vi "GDFeventTypeHandler.vi"(1 "EventTypeCode":u16) -> (0 "EventTypeString":string)   [LabVIEW 2016, in "GDF File Reader.lvlib"]
uses:
  GDF File Reader.lvlib
panel:
  # "This VI is a part of BCI Design library, http://www.ru-bci.org \nCopyright © 2020, Sotnikov Peter, All rights reserved. License: CC BY-NC 4.0"
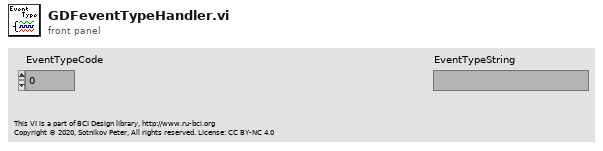
[diagram p1: front panel]
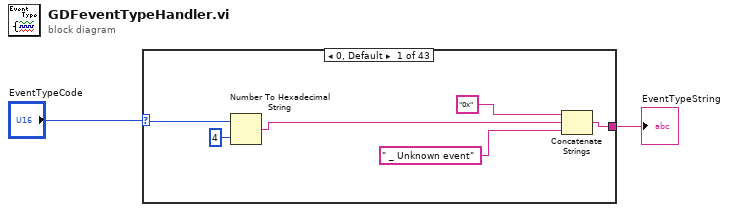
[diagram p0: block diagram]
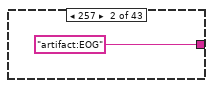
[diagram p2: hidden frame]
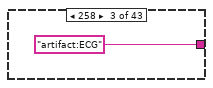
[diagram p3: hidden frame]
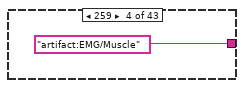
[diagram p4: hidden frame]
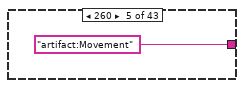
[diagram p5: hidden frame]
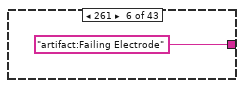
[diagram p6: hidden frame]
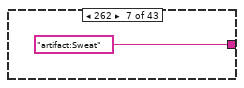
[diagram p7: hidden frame]
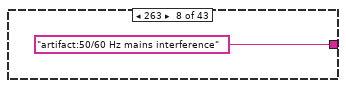
[diagram p8: hidden frame]
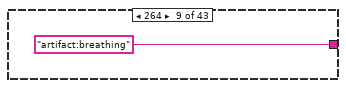
[diagram p9: hidden frame]
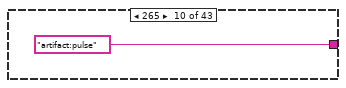
[diagram p10: hidden frame]
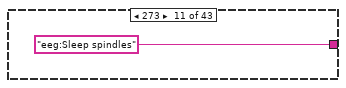
[diagram p11: hidden frame]
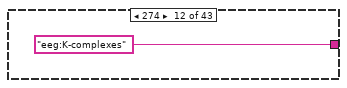
[diagram p12: hidden frame]
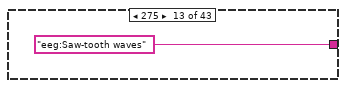
[diagram p13: hidden frame]
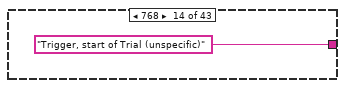
[diagram p14: hidden frame]
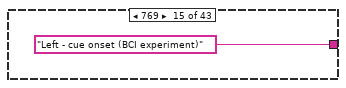
[diagram p15: hidden frame]
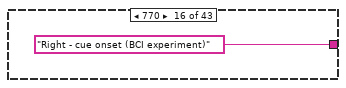
[diagram p16: hidden frame]
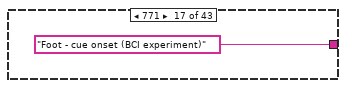
[diagram p17: hidden frame]
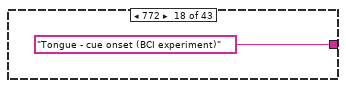
[diagram p18: hidden frame]
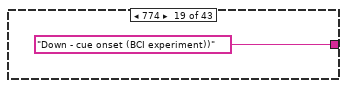
[diagram p19: hidden frame]
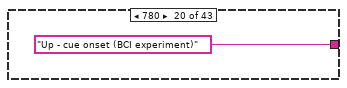
[diagram p20: hidden frame]
diagram:
  n1 = case shown="0, Default" "EventTypeCode" {
    selector: "EventTypeCode" -> [w7 _ _ _ _ _ _ _ _ _ _ _ _ _ _ _ _ _ _ _ _ _ _ _ _ _ _ _ _ _ _ _ _ _ _ _ _ _ _ _ _ _ _]
    tunnel: [w6 "artifact:EOG" "artifact:ECG" "artifact:EMG/Muscle" "artifact:Movement" "artifact:Failing Electrode" "artifact:Sweat" "artifact:50/60 Hz mains interference" "artifact:breathing" "artifact:pulse" "eeg:Sleep spindles" "eeg:K-complexes" "eeg:Saw-tooth waves" "Trigger, start of Trial (unspecific)" "Left - cue onset (BCI experiment)" "Right - cue onset (BCI experiment)" "Foot - cue onset (BCI experiment)" "Tongue - cue onset (BCI experiment)" "Down - cue onset (BCI experiment))" "Up - cue onset (BCI experiment)" "Feedback (continuous) - onset (BCI experiment)" "Feedback (discrete) - onset (BCI experiment)" "Beep (accustic stimulus, BCI experiment)" "Cross on screen (BCI experiment)" "Rejection of whole trial" "Obstructive Apnea/Hypopnea Event (OAHE)" "Respiratory Effort Related Arousal (RERA)" "Central Apnea/Hypopnea Event (CAHE)" "Cheyne-Stokes Breathing (CSB)" "Sleep Hypoventilation" "Wake" "Stage 1" "Stage 2" "Stage 3" "Stage 4" "REM" "ecg:Fiducial point of QRS complex" "ecg:P-wave" "ecg:Q-point" "ecg:R-point" "ecg:S-point" "ecg:T-point" "ecg:U-wave"] -> w1
    frame 0, Default {
      n2 = Number To Hexadecimal String(1:i16 4 ("width (-)"), 2:w7) -> (0:w5:string)
      n3 = Concatenate Strings("0x" ("string"), w5, " _ Unknown event") -> (w6:string)
    }
    frame 257 {
    }
    frame 258 {
    }
    frame 259 {
    }
    frame 260 {
    }
    frame 261 {
    }
    frame 262 {
    }
    frame 263 {
    }
    frame 264 {
    }
    frame 265 {
    }
    frame 273 {
    }
    frame 274 {
    }
    frame 275 {
    }
    frame 768 {
    }
    frame 769 {
    }
    frame 770 {
    }
    frame 771 {
    }
    frame 772 {
    }
    frame 774 {
    }
    frame 780 {
    }
    frame 781 {
    }
    frame 782 {
    }
    frame 785 {
    }
    frame 786 {
    }
    frame 1023 {
    }
    frame 1025 {
    }
    frame 1026 {
    }
    frame 1027 {
    }
    frame 1028 {
    }
    frame 1029 {
    }
    frame 1040 {
    }
    frame 1041 {
    }
    frame 1042 {
    }
    frame 1043 {
    }
    frame 1044 {
    }
    frame 1045 {
    }
    frame 1281 {
    }
    frame 1282 {
    }
    frame 1283 {
    }
    frame 1284 {
    }
    frame 1285 {
    }
    frame 1286 {
    }
    frame 1287 {
    }
  }
  "EventTypeString" <- w1
